vi "Logger-Start.vi"(0 "Folder":path, 5 "Name":string, 7 "Level":T1=enum."Info", 9 "Retain (days)":i32=14, 11 "Length":i32=10000) -> (15 "error out":errorcluster)   [LabVIEW 2020]
uses:
  Typedefs/Logger-Level.ctl
  <vilib>/Utility/sysdir.llb/System Directory Type.ctl
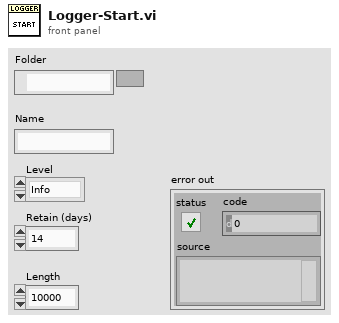
[diagram p1: front panel]
types:
  T1 = typedef "Logger-Level.ctl" = enum16{"Debug", "TCP", "Info", "Warning", "Error", "Critical"}
  T2 = typedef "System Directory Type.ctl" = i32
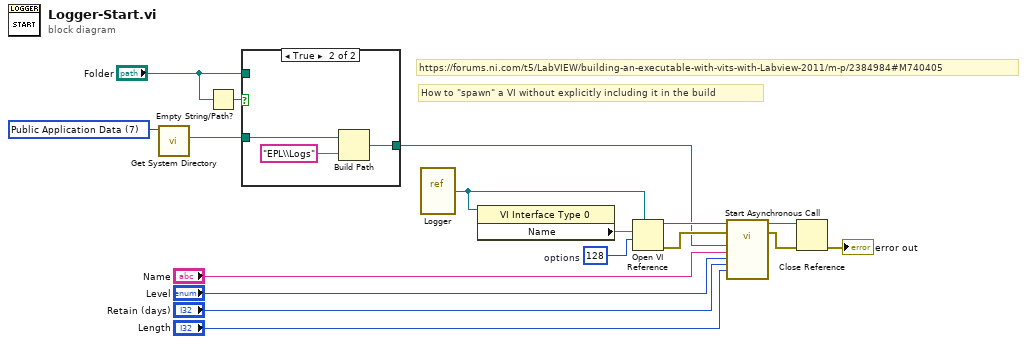
[diagram p0: block diagram]
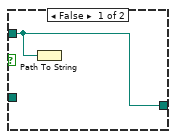
[diagram p2: hidden frame]
diagram:
  w11 = 128  # options
  w17 = T2 7 items=["User Home"=0, "User Desktop"=1, "User Documents"=2, "User Application Data"=3, "User Preferences"=4, "User Temporary"=5, "Public Documents"=6, "Public Application Data"=7, "Public Preferences"=8, "Public Cache"=13, "System Core Libraries"=9, "System Installed Libraries"=10, "Application Files"=11, "Boot Volume Root"=12] ("system directory type")
  # "How to \"spawn\" a VI without explicitly including it in the build"
  # "https://forums.ni.com/t5/LabVIEW/building-an-executable-with-vits-with-Labview-2011/m-p/2384984#M740405"
  n1 = call <vilib>:"Get System Directory.vi"("system directory type"=w17) -> ("system directory"=w15:path)  [unwired: 10 in]
  n2 = Empty String/Path?(string/path="Folder") -> (empty?=w16:bool)
  n3 = case shown="True" w16 {
    tunnel: w15 -> [_ w21]
    tunnel: [w18 w19] -> w6
    tunnel: "Folder" -> [w18 _]
    frame False {
      n4 = Path To String(path=w18) -> ()  [unwired: 1 out]
    }
    frame True {
      n5 = Build Path(base path=w21, name or relative path="EPL\\Logs") -> (appended path=w19:path)
    }
  }
  n6 = vi-ref "Logger.vi"() -> (w13:refnum<vi>)
  n7 = property class="VI Interface Type 0"(reference=w13) -> ("Name"=w12:string)  [unwired: 1 in, 2 out]
  n8 = Open VI Reference(type specifier VI Refnum (for type only)=w13, vi path=w12, options=w11) -> (vi reference=w10:refnum<vi>, error out=w9:errorcluster)  [unwired: 3 in]
  n9 = call-by-ref "Start Asynchronous Call"(reference=w10, error in=w9, "Folder"=w6, "Name"="Name", "Level"="Level", "Retain (days)"="Retain (days)", "Length"="Length") -> (reference out=w8:refnum<vi>, error out=w7:errorcluster)  [unwired: 11 in]
  n10 = Close Reference(reference=w8, error in (no error)=w7) -> (error out=→"error out":errorcluster)
